vi "MFLI find module handle.vi"(10 "module Id":T2 items=["sweep", "scopeModule", "dataAcquisitionModule", "pidAdvisor", "awgModule", "impedanceModule", "multiDeviceSyncModule", "zoomFFT", "trigger", "deviceSettings", "record", "precompensationAdvisor"], 11 "ModuleHandles":T1[](array[typedef]) {"ModHandle" format="0x%08x"; "Conn" format="0x%08x"}) -> (1 "was found":bool, 2 "index":i32, 3 "ziModHandle out":T1 {"ModHandle" format="0x%08x"; "Conn" format="0x%08x"})   [LabVIEW 2024, in "Lock-in module.lvlib"]
uses:
  Lock-in module.lvlib
  <instrlib>/Zurich Instruments LabOne/Public/Modules/ziTypeModEnum.ctl
  <instrlib>/Zurich Instruments LabOne/Public/Modules/ziTypeModHandle.ctl
  <instrlib>/Zurich Instruments LabOne/Zurich Instruments LabOne.lvlib
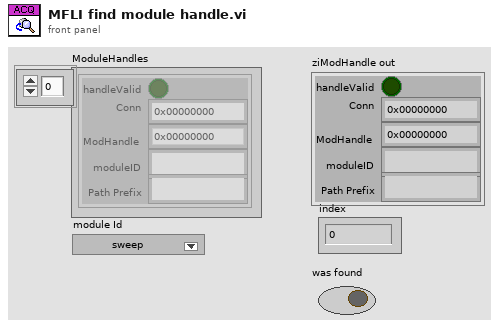
[diagram p1: front panel]
types:
  T1 = typedef "Zurich Instruments LabOne.lvlib/ziTypeModHandle.ctl" = cluster{"handleValid":bool, "Conn":u64, "ModHandle":u64, "moduleID":string, "Path Prefix":string}
  T2 = typedef "Zurich Instruments LabOne.lvlib/ziTypeModEnum.ctl" = u16
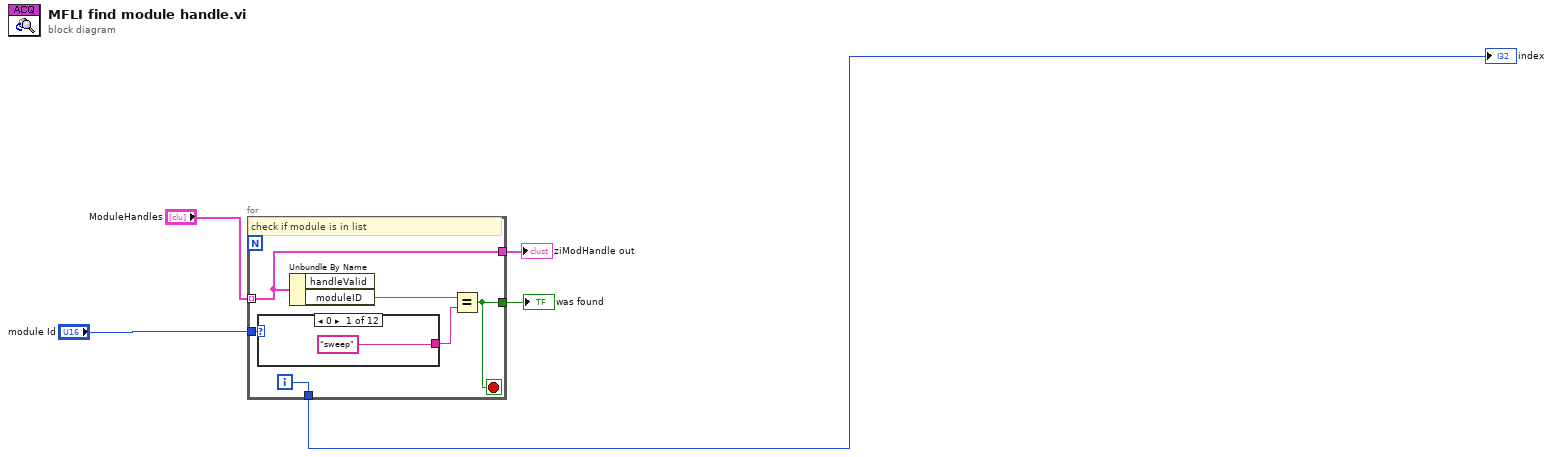
[diagram p0: block diagram]
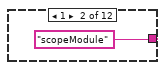
[diagram p2: hidden frame]
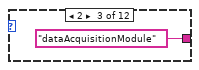
[diagram p3: hidden frame]
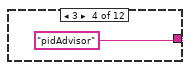
[diagram p4: hidden frame]
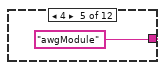
[diagram p5: hidden frame]
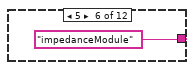
[diagram p6: hidden frame]
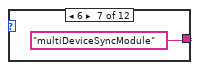
[diagram p7: hidden frame]
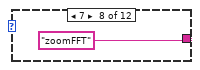
[diagram p8: hidden frame]
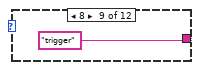
[diagram p9: hidden frame]
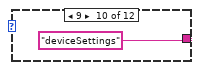
[diagram p10: hidden frame]
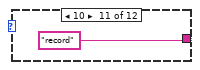
[diagram p11: hidden frame]
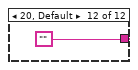
[diagram p12: hidden frame]
diagram:
  n1 = for {
    tunnel: "ModuleHandles" -> [w6] mode=indexing
    tunnel: "module Id" -> [w9]
    tunnel: [w8] -> w2
    tunnel: [w7] -> w5
    tunnel: [w6] -> w3
    i -> [w8]
    stop <- w7 stop-if-true
    # "check if module is in list"
    n2 = case shown="0" w9 {
      tunnel: ["sweep" "scopeModule" "dataAcquisitionModule" "pidAdvisor" "awgModule" "impedanceModule" "multiDeviceSyncModule" "zoomFFT" "trigger" "deviceSettings" "record" ""] -> w10
      frame 0 {
      }
      frame 1 {
      }
      frame 2 {
      }
      frame 3 {
      }
      frame 4 {
      }
      frame 5 {
      }
      frame 6 {
      }
      frame 7 {
      }
      frame 8 {
      }
      frame 9 {
      }
      frame 10 {
      }
      frame 20, Default {
      }
    }
    n3 = Unbundle By Name(w6) -> ("moduleID"=w11:string)  [unwired: 1 out]
    n4 = Equal?(x=w11, y=w10) -> (x = y?=w7:bool)
  }
  "was found" <- w5
  "ziModHandle out" <- w3
  "index" <- w2
